vi "Arduino read multiple 10times resolution.vi"(6 "main loop iteration number":i32, 8 "arduino addresses in":T2, 10 "arduinos on?":bool) -> (1 "arduino addresses out":T2, 2 "unfiltered and mean of median filtered freq out":T1, 3 "arduinos on":bool)   [LabVIEW 2014]
uses:
  <vilib>/Analysis/baseanly.llb/Mean (DBL).vi
  <vilib>/Analysis/NI_AALBase.lvlib
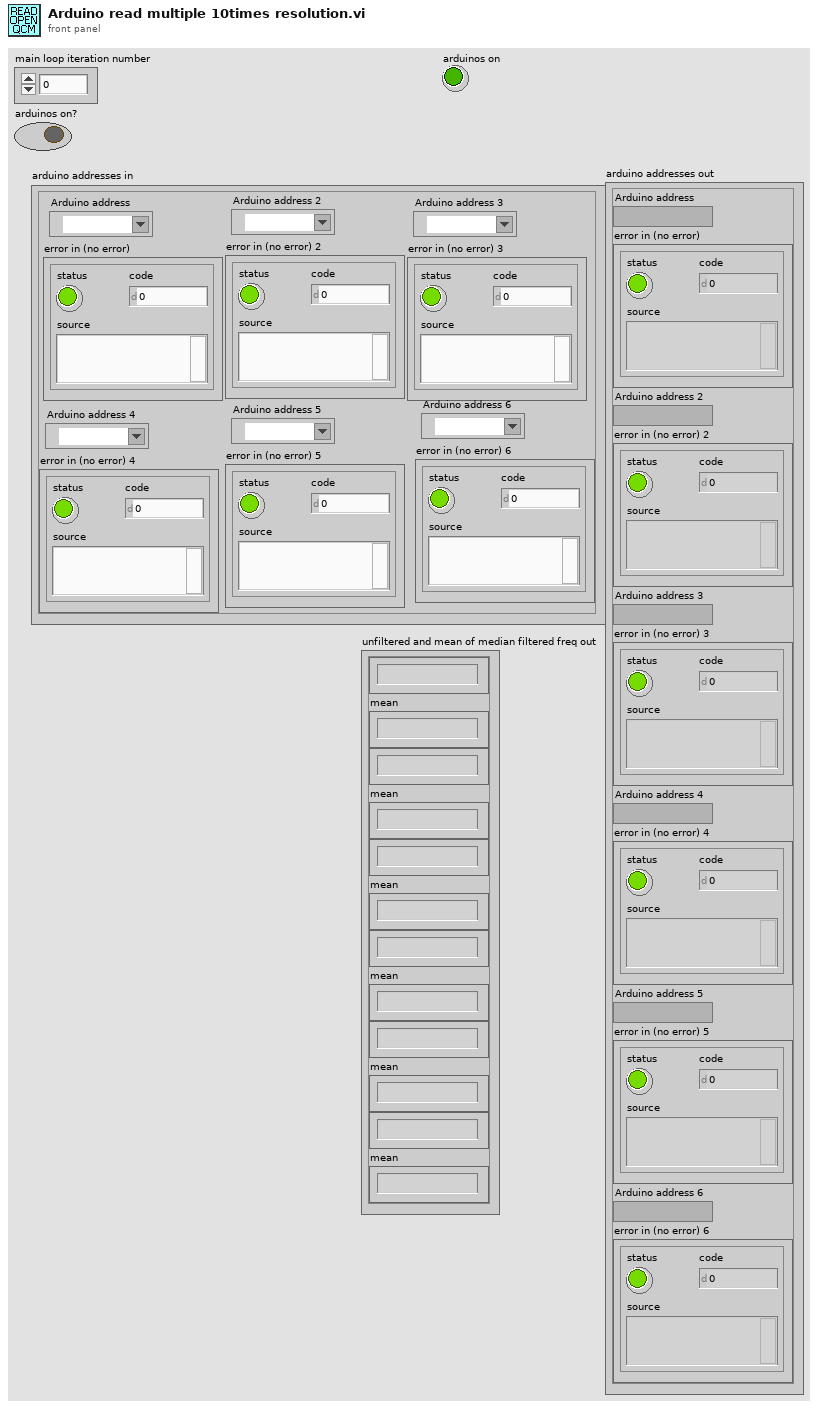
[diagram p1: front panel]
types:
  T1 = cluster{"String":string, "mean":string, "String":string, "mean":string, "String":string, "mean":string, "String":string, "mean":string, "String":string, "mean":string, "String":string, "mean":string}
  T2 = cluster{"Arduino address":refnum<visa-resource-name>, "error in (no error)":errorcluster, "Arduino address 2":refnum<visa-resource-name>, "error in (no error) 2":errorcluster, "Arduino address 3":refnum<visa-resource-name>, "error in (no error) 3":errorcluster, "Arduino address 4":refnum<visa-resource-name>, "error in (no error) 4":errorcluster, "Arduino address 5":refnum<visa-resource-name>, "error in (no error) 5":errorcluster, "Arduino address 6":refnum<visa-resource-name>, "error in (no error) 6":errorcluster}
  T3 = cluster{string, "mean":string, string, "mean":string, string, "mean":string, string, "mean":string, string, "mean":string, string, "mean":string}
  T4 = cluster{dbl, "mean":dbl, dbl, "mean":dbl, dbl, "mean":dbl, dbl, "mean":dbl, dbl, "mean":dbl, dbl, "mean":dbl}
  T5 = cluster{"Arduino address":refnum<visa-resource-name>, "error out":errorcluster, "Arduino address 2":refnum<visa-resource-name>, "error out":errorcluster, "Arduino address 3":refnum<visa-resource-name>, "error out":errorcluster, "Arduino address 4":refnum<visa-resource-name>, "error out":errorcluster, "Arduino address 5":refnum<visa-resource-name>, "error out":errorcluster, "Arduino address 6":refnum<visa-resource-name>, "error out":errorcluster}
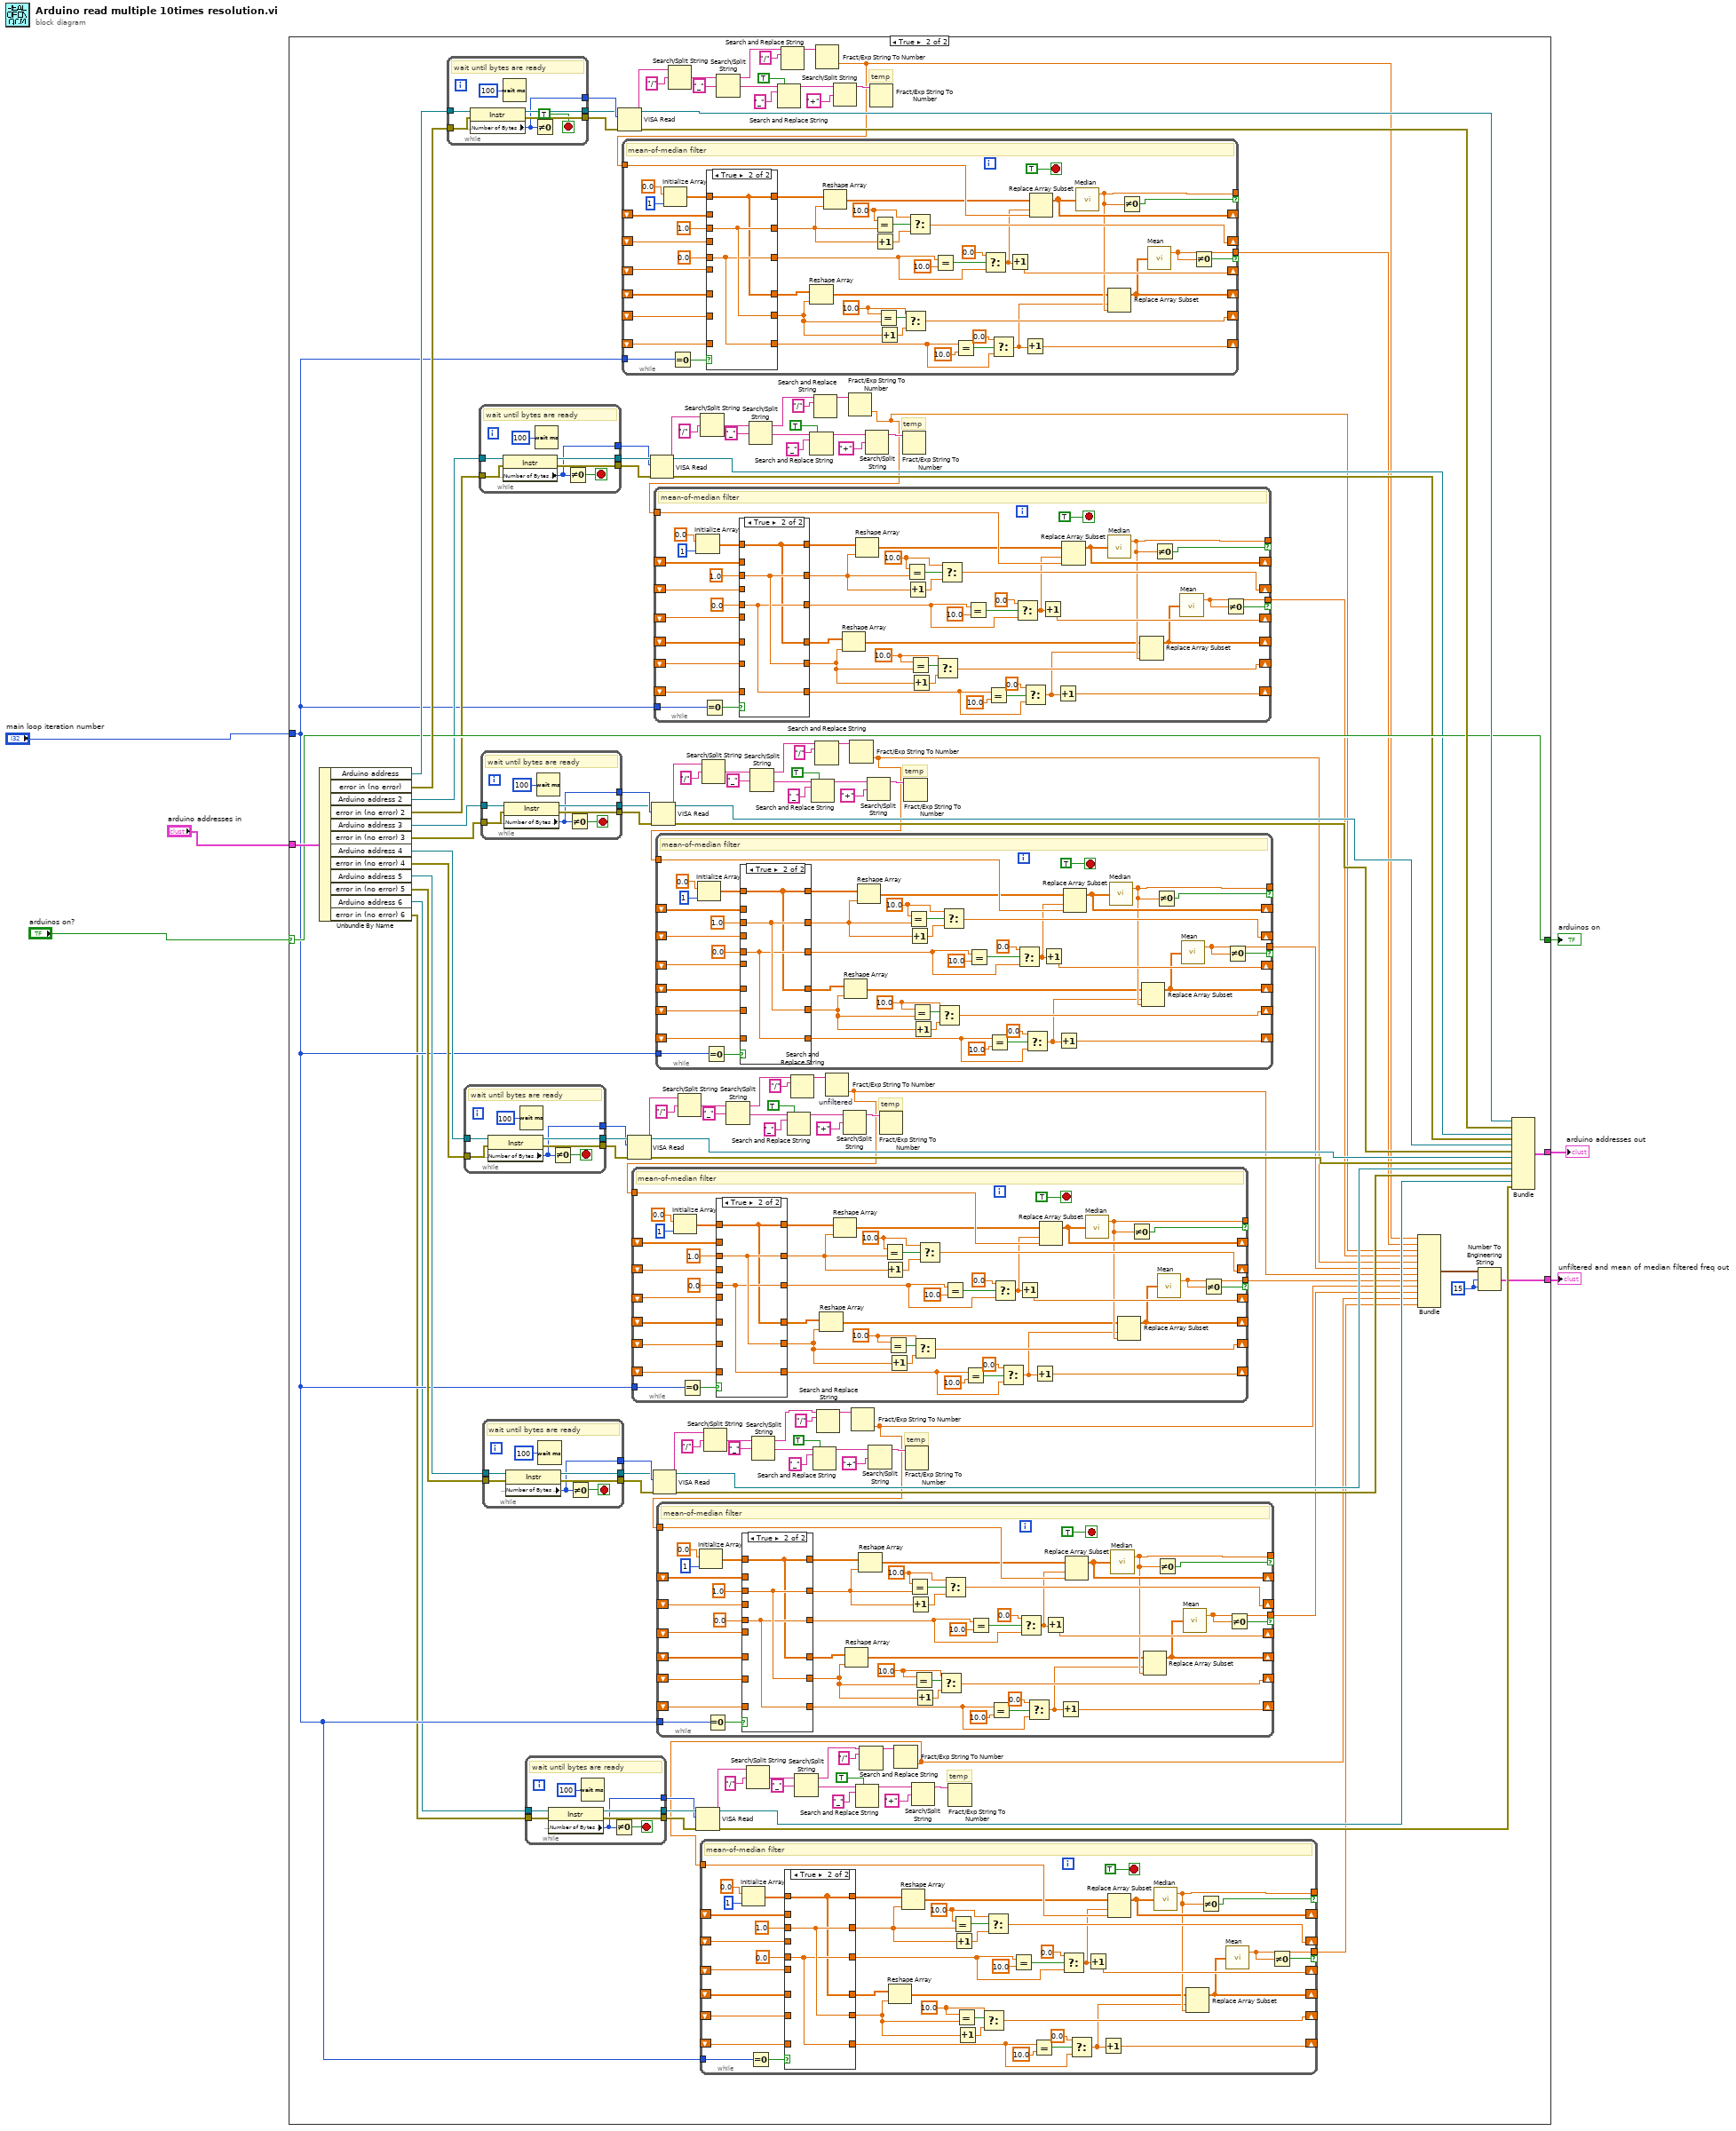
[diagram p0: block diagram]
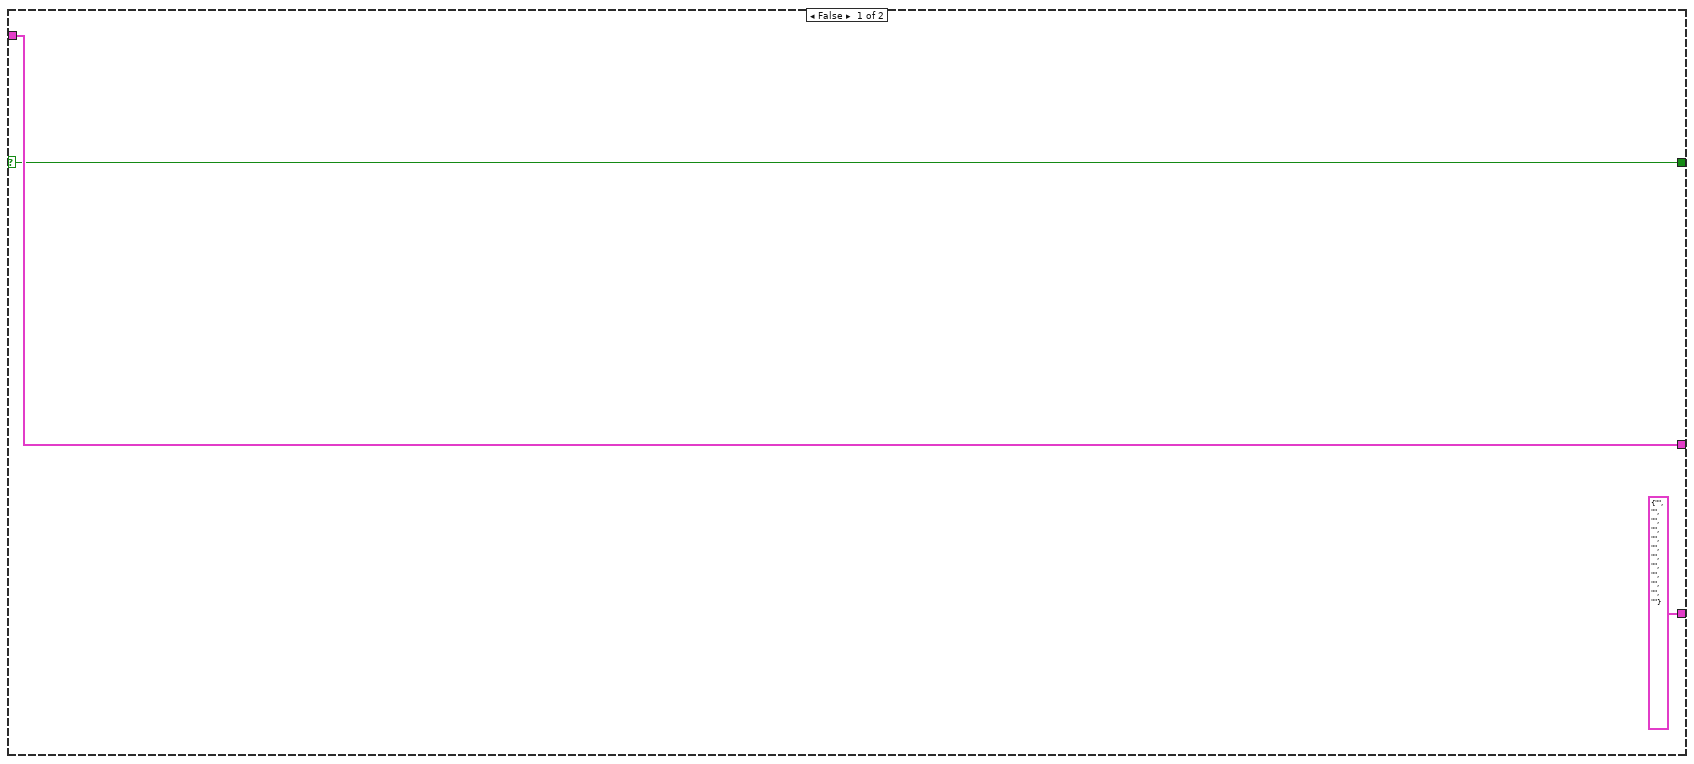
[diagram p2: hidden frame]
diagram:
  n1 = case shown="True" "arduinos on?" {
    selector: "arduinos on?" -> [w8 w126]
    tunnel: "main loop iteration number" -> [_ w31]
    tunnel: "arduino addresses in" -> [w9 w132]
    tunnel: [w9 w127] -> w2
    tunnel: [w8 w126] -> w3
    tunnel: [T3 {"", "mean"="", "", "mean"="", "", "mean"="", "", "mean"="", "", "mean"="", "", "mean"=""} w22] -> w1
    frame False {
    }
    frame True {
      w24 = i16 15 ("width (-)")
      # "temp"
      # "temp"
      # "temp"
      # "temp"
      # "temp"
      # "temp"
      n2 = Unbundle By Name(w132) -> ("Arduino address"=w131:refnum<visa-resource-name>, "error in (no error)"=w130:errorcluster, "Arduino address 2"=w109:refnum<visa-resource-name>, "error in (no error) 2"=w108:errorcluster, "Arduino address 3"=w89:refnum<visa-resource-name>, "error in (no error) 3"=w88:errorcluster, "Arduino address 4"=w69:refnum<visa-resource-name>, "error in (no error) 4"=w68:errorcluster, "Arduino address 5"=w51:refnum<visa-resource-name>, "error in (no error) 5"=w50:errorcluster, "Arduino address 6"=w30:refnum<visa-resource-name>, "error in (no error) 6"=w29:errorcluster)
      n3 = while {
        tunnel: w130 -> [w469]
        tunnel: w131 -> [w470]
        tunnel: [w468] -> w134
        tunnel: [w467] -> w133
        tunnel: [w466] -> w135
        stop <- TRUE stop-if-true
        # "wait until bytes are ready"
        n4 = property class="Instr"(reference=w470, error in=w469) -> (reference out=w467:refnum<visa-resource-name>, error out=w468:errorcluster, "Serial Settings:Number of Bytes at Serial Port"=w466:u32)
        n5 = Wait (ms)(milliseconds to wait=u32 100) -> ()  [unwired: 1 out]
        n6 = Not Equal To 0?(x=w466) -> ()  [unwired: 1 out]
      }
      n7 = while {
        tunnel: w68 -> [w280]
        tunnel: w69 -> [w281]
        tunnel: [w279] -> w84
        tunnel: [w278] -> w85
        tunnel: [w277] -> w83
        stop <- w275 stop-if-true
        # "wait until bytes are ready"
        n8 = property class="Instr"(reference=w281, error in=w280) -> (reference out=w278:refnum<visa-resource-name>, error out=w279:errorcluster, "Serial Settings:Number of Bytes at Serial Port"=w277:u32)
        n9 = Wait (ms)(milliseconds to wait=u32 100) -> ()  [unwired: 1 out]
        n10 = Not Equal To 0?(x=w277) -> (x != 0?=w275:bool)
      }
      n11 = while {
        tunnel: w108 -> [w406]
        tunnel: w109 -> [w407]
        tunnel: [w405] -> w124
        tunnel: [w404] -> w125
        tunnel: [w403] -> w123
        stop <- w401 stop-if-true
        # "wait until bytes are ready"
        n12 = property class="Instr"(reference=w407, error in=w406) -> (reference out=w404:refnum<visa-resource-name>, error out=w405:errorcluster, "Serial Settings:Number of Bytes at Serial Port"=w403:u32)
        n13 = Wait (ms)(milliseconds to wait=u32 100) -> ()  [unwired: 1 out]
        n14 = Not Equal To 0?(x=w403) -> (x != 0?=w401:bool)
      }
      n15 = while {
        tunnel: w88 -> [w343]
        tunnel: w89 -> [w344]
        tunnel: [w342] -> w91
        tunnel: [w341] -> w90
        tunnel: [w340] -> w92
        stop <- w338 stop-if-true
        # "wait until bytes are ready"
        n16 = property class="Instr"(reference=w344, error in=w343) -> (reference out=w341:refnum<visa-resource-name>, error out=w342:errorcluster, "Serial Settings:Number of Bytes at Serial Port"=w340:u32)
        n17 = Wait (ms)(milliseconds to wait=u32 100) -> ()  [unwired: 1 out]
        n18 = Not Equal To 0?(x=w340) -> (x != 0?=w338:bool)
      }
      n19 = while {
        tunnel: w51 -> [w218]
        tunnel: [w217] -> w53
        tunnel: [w216] -> w52
        tunnel: [w215] -> w54
        tunnel: w50 -> [w212]
        stop <- w213 stop-if-true
        # "wait until bytes are ready"
        n20 = property class="Instr"(reference=w218, error in=w212) -> (reference out=w216:refnum<visa-resource-name>, error out=w217:errorcluster, "Serial Settings:Number of Bytes at Serial Port"=w215:u32)
        n21 = Wait (ms)(milliseconds to wait=u32 100) -> ()  [unwired: 1 out]
        n22 = Not Equal To 0?(x=w215) -> (x != 0?=w213:bool)
      }
      n23 = while {
        tunnel: w30 -> [w155]
        tunnel: [w154] -> w46
        tunnel: [w153] -> w47
        tunnel: [w152] -> w45
        tunnel: w29 -> [w149]
        stop <- w150 stop-if-true
        # "wait until bytes are ready"
        n24 = property class="Instr"(reference=w155, error in=w149) -> (reference out=w153:refnum<visa-resource-name>, error out=w154:errorcluster, "Serial Settings:Number of Bytes at Serial Port"=w152:u32)
        n25 = Wait (ms)(milliseconds to wait=u32 100) -> ()  [unwired: 1 out]
        n26 = Not Equal To 0?(x=w152) -> (x != 0?=w150:bool)
      }
      n27 = VISA Read(VISA resource name=w133, byte count=w135, error in (no error)=w134) -> (VISA resource name out=w129:refnum<visa-resource-name>, read buffer=w148:string, error out=w128:errorcluster)  [unwired: 1 out]
      n28 = VISA Read(VISA resource name=w85, byte count=w83, error in (no error)=w84) -> (VISA resource name out=w67:refnum<visa-resource-name>, read buffer=w70:string, error out=w66:errorcluster)  [unwired: 1 out]
      n29 = VISA Read(VISA resource name=w125, byte count=w123, error in (no error)=w124) -> (VISA resource name out=w106:refnum<visa-resource-name>, read buffer=w110:string, error out=w107:errorcluster)  [unwired: 1 out]
      n30 = VISA Read(VISA resource name=w90, byte count=w92, error in (no error)=w91) -> (VISA resource name out=w87:refnum<visa-resource-name>, read buffer=w105:string, error out=w86:errorcluster)  [unwired: 1 out]
      n31 = VISA Read(VISA resource name=w52, byte count=w54, error in (no error)=w53) -> (VISA resource name out=w49:refnum<visa-resource-name>, read buffer=w65:string, error out=w48:errorcluster)  [unwired: 1 out]
      n32 = Search/Split String(string=w148, search string/char (-)="/") -> (match + rest of string=w141:string)  [unwired: 1 in, 2 out]
      n33 = Search/Split String(string=w70, search string/char (-)="/") -> (match + rest of string=w77:string)  [unwired: 1 in, 2 out]
      n34 = VISA Read(VISA resource name=w47, byte count=w45, error in (no error)=w46) -> (VISA resource name out=w26:refnum<visa-resource-name>, read buffer=w34:string, error out=w25:errorcluster)  [unwired: 1 out]
      n35 = Search/Split String(string=w110, search string/char (-)="/") -> (match + rest of string=w117:string)  [unwired: 1 in, 2 out]
      n36 = Search/Split String(string=w105, search string/char (-)="/") -> (match + rest of string=w98:string)  [unwired: 1 in, 2 out]
      n37 = Search/Split String(string=w65, search string/char (-)="/") -> (match + rest of string=w59:string)  [unwired: 1 in, 2 out]
      n38 = Search/Split String(string=w141, search string/char (-)="_") -> (substring before match=w147:string, match + rest of string=w142:string)  [unwired: 1 in, 1 out]
      n39 = Search/Split String(string=w77, search string/char (-)="_") -> (substring before match=w71:string, match + rest of string=w76:string)  [unwired: 1 in, 1 out]
      n40 = Search/Split String(string=w34, search string/char (-)="/") -> (match + rest of string=w40:string)  [unwired: 1 in, 2 out]
      n41 = Search/Split String(string=w117, search string/char (-)="_") -> (substring before match=w111:string, match + rest of string=w116:string)  [unwired: 1 in, 1 out]
      n42 = Search/Split String(string=w98, search string/char (-)="_") -> (substring before match=w104:string, match + rest of string=w99:string)  [unwired: 1 in, 1 out]
      n43 = Search/Split String(string=w59, search string/char (-)="_") -> (substring before match=w33:string, match + rest of string=w60:string)  [unwired: 1 in, 1 out]
      n44 = Search and Replace String(replace all?=TRUE ("replace all? (F)"), input string=w142, search string="_") -> (result string=w136:string)  [unwired: 5 in, 3 out]
      n45 = Search and Replace String(input string=w147, search string="/" ("replace string (\"\")")) -> (result string=w138:string)  [unwired: 6 in, 3 out]
      n46 = Search and Replace String(replace all?=TRUE ("replace all? (F)"), input string=w76, search string="_") -> (result string=w82:string)  [unwired: 5 in, 3 out]
      n47 = Search and Replace String(input string=w71, search string="/" ("replace string (\"\")")) -> (result string=w80:string)  [unwired: 6 in, 3 out]
      n48 = Search/Split String(string=w40, search string/char (-)="_") -> (substring before match=w28:string, match + rest of string=w39:string)  [unwired: 1 in, 1 out]
      n49 = Search and Replace String(replace all?=TRUE ("replace all? (F)"), input string=w116, search string="_") -> (result string=w122:string)  [unwired: 5 in, 3 out]
      n50 = Search and Replace String(replace all?=TRUE ("replace all? (F)"), input string=w99, search string="_") -> (result string=w93:string)  [unwired: 5 in, 3 out]
      n51 = Search and Replace String(replace all?=TRUE ("replace all? (F)"), input string=w60, search string="_") -> (result string=w55:string)  [unwired: 5 in, 3 out]
      n52 = Search and Replace String(input string=w111, search string="/" ("replace string (\"\")")) -> (result string=w120:string)  [unwired: 6 in, 3 out]
      n53 = Search and Replace String(input string=w104, search string="/" ("replace string (\"\")")) -> (result string=w95:string)  [unwired: 6 in, 3 out]
      n54 = Fract/Exp String To Number(string=w138) -> (number=w21:dbl)  [unwired: 3 in, 1 out]
      n55 = while {
        shift-right: [w509] -> _
        shift-left: _ -> [w487]
        shift-right: [w517] -> _
        shift-left: _ -> [w480]
        shift-right: [w506] -> _
        shift-left: _ -> [w477]
        shift-right: [w516] -> _
        shift-left: _ -> [w473]
        shift-right: [w515] -> _
        shift-left: _ -> [w484]
        tunnel: w21 -> [w512]
        tunnel: w31 -> [w489]
        tunnel: [w508] -> w15 if=w511
        tunnel: [w505] -> _ if=w504
        shift-right: [w507] -> _
        shift-left: _ -> [w475]
        stop <- TRUE stop-if-true
        w490 = 10.0 ("t")
        w482 = 10.0 ("y")
        # "mean-of-median filter"
        n56 = Initialize Array(0.0 ("element"), 1 ("dimension size")) -> (w478:dbl[])
        n57 = Equal To 0?(x=w489) -> (x = 0?=w488:bool)
        n58 = case shown="True" w488 {
          tunnel: w478 -> [_ w524]
          tunnel: w487 -> [w523 _]
          tunnel: [w523 w524] -> w486
          tunnel: 1.0 ("t") -> [_ w526]
          tunnel: w484 -> [w522 _]
          tunnel: [w522 w526] -> w483
          tunnel: 0.0 ("t") -> [_ w525]
          tunnel: [w521 w525] -> w479
          tunnel: w480 -> [w521 _]
          tunnel: [w520 w524] -> w476
          tunnel: w477 -> [w520 _]
          tunnel: [w519 w526] -> w474
          tunnel: w475 -> [w519 _]
          tunnel: w473 -> [w518 _]
          tunnel: [w518 w525] -> w472
          frame False {
          }
          frame True {
          }
        }
        n59 = Reshape Array(w476, w474) -> (w471:dbl[])
        n60 = Reshape Array(w486, w483) -> (w497:dbl[])
        n61 = Equal?(x=w482, y=w483) -> (x = y?=w496:bool)
        n62 = Increment(x=w483) -> (x+1=w495:dbl)
        n63 = Equal?(x=w490, y=w474) -> (x = y?=w493:bool)
        n64 = Increment(x=w474) -> (x+1=w492:dbl)
        n65 = Select(t=w490, s=w493, f=w492) -> (s? t:f=w507:dbl)
        n66 = Select(t=w482, s=w496, f=w495) -> (s? t:f=w515:dbl)
        n67 = Equal?(x=w479, y=10.0) -> (x = y?=w503:bool)
        n68 = Equal?(x=w472, y=10.0) -> (x = y?=w500:bool)
        n69 = Select(t=0.0, s=w503, f=w479) -> (s? t:f=w491:dbl)
        n70 = Select(t=0.0, s=w500, f=w472) -> (s? t:f=w499:dbl)
        n71 = Increment(x=w491) -> (x+1=w517:dbl)
        n72 = Increment(x=w499) -> (x+1=w516:dbl)
        n73 = Replace Array Subset(array=w497, new element=w512, index=w491) -> (w509:dbl[])
        n74 = call <vilib>:"Median.vi"("X"=w509) -> ("median"=w505:dbl)  [unwired: 1 out]
        n75 = Replace Array Subset(array=w471, new element=w505, index=w499) -> (w506:dbl[])
        n76 = Not Equal To 0?(x=w505) -> (x != 0?=w504:bool)
        n77 = call-poly <vilib>:"Mean.vi"("X"=w506) -> ("mean"=w508:dbl)  [unwired: 1 out]
        n78 = Not Equal To 0?(x=w508) -> (x != 0?=w511:bool)
      }
      n79 = Search and Replace String(input string=w33, search string="/" ("replace string (\"\")")) -> (result string=w32:string)  [unwired: 6 in, 3 out]
      n80 = Fract/Exp String To Number "unfiltered"(string=w80) -> (number=w18:dbl)  [unwired: 3 in, 1 out]
      n81 = while {
        shift-right: [w320] -> _
        shift-left: _ -> [w298]
        shift-right: [w328] -> _
        shift-left: _ -> [w291]
        shift-right: [w317] -> _
        shift-left: _ -> [w288]
        shift-right: [w327] -> _
        shift-left: _ -> [w284]
        shift-right: [w326] -> _
        shift-left: _ -> [w295]
        tunnel: w18 -> [w323]
        tunnel: w31 -> [w300]
        tunnel: [w319] -> w12 if=w322
        tunnel: [w316] -> _ if=w315
        shift-right: [w318] -> _
        shift-left: _ -> [w286]
        stop <- TRUE stop-if-true
        w301 = 10.0 ("t")
        w293 = 10.0 ("y")
        # "mean-of-median filter"
        n82 = Initialize Array(0.0 ("element"), 1 ("dimension size")) -> (w289:dbl[])
        n83 = Equal To 0?(x=w300) -> (x = 0?=w299:bool)
        n84 = case shown="True" w299 {
          tunnel: w289 -> [_ w335]
          tunnel: w298 -> [w334 _]
          tunnel: [w334 w335] -> w297
          tunnel: 1.0 ("t") -> [_ w337]
          tunnel: w295 -> [w333 _]
          tunnel: [w333 w337] -> w294
          tunnel: 0.0 ("t") -> [_ w336]
          tunnel: [w332 w336] -> w290
          tunnel: w291 -> [w332 _]
          tunnel: [w331 w335] -> w287
          tunnel: w288 -> [w331 _]
          tunnel: [w330 w337] -> w285
          tunnel: w286 -> [w330 _]
          tunnel: w284 -> [w329 _]
          tunnel: [w329 w336] -> w283
          frame False {
          }
          frame True {
          }
        }
        n85 = Reshape Array(w287, w285) -> (w282:dbl[])
        n86 = Reshape Array(w297, w294) -> (w308:dbl[])
        n87 = Equal?(x=w293, y=w294) -> (x = y?=w307:bool)
        n88 = Increment(x=w294) -> (x+1=w306:dbl)
        n89 = Equal?(x=w301, y=w285) -> (x = y?=w304:bool)
        n90 = Increment(x=w285) -> (x+1=w303:dbl)
        n91 = Select(t=w301, s=w304, f=w303) -> (s? t:f=w318:dbl)
        n92 = Select(t=w293, s=w307, f=w306) -> (s? t:f=w326:dbl)
        n93 = Equal?(x=w290, y=10.0) -> (x = y?=w314:bool)
        n94 = Equal?(x=w283, y=10.0) -> (x = y?=w311:bool)
        n95 = Select(t=0.0, s=w314, f=w290) -> (s? t:f=w302:dbl)
        n96 = Select(t=0.0, s=w311, f=w283) -> (s? t:f=w310:dbl)
        n97 = Increment(x=w302) -> (x+1=w328:dbl)
        n98 = Increment(x=w310) -> (x+1=w327:dbl)
        n99 = Replace Array Subset(array=w308, new element=w323, index=w302) -> (w320:dbl[])
        n100 = call <vilib>:"Median.vi"("X"=w320) -> ("median"=w316:dbl)  [unwired: 1 out]
        n101 = Replace Array Subset(array=w282, new element=w316, index=w310) -> (w317:dbl[])
        n102 = Not Equal To 0?(x=w316) -> (x != 0?=w315:bool)
        n103 = call-poly <vilib>:"Mean.vi"("X"=w317) -> ("mean"=w319:dbl)  [unwired: 1 out]
        n104 = Not Equal To 0?(x=w319) -> (x != 0?=w322:bool)
      }
      n105 = Search/Split String(string=w136, search string/char (-)="+") -> (substring before match=w145:string)  [unwired: 1 in, 2 out]
      n106 = Search/Split String(string=w82, search string/char (-)="+") -> (substring before match=w73:string)  [unwired: 1 in, 2 out]
      n107 = Fract/Exp String To Number(string=w120) -> (number=w20:dbl)  [unwired: 3 in, 1 out]
      n108 = while {
        shift-right: [w446] -> _
        shift-left: _ -> [w424]
        shift-right: [w454] -> _
        shift-left: _ -> [w417]
        shift-right: [w443] -> _
        shift-left: _ -> [w414]
        shift-right: [w453] -> _
        shift-left: _ -> [w410]
        shift-right: [w452] -> _
        shift-left: _ -> [w421]
        tunnel: w20 -> [w449]
        tunnel: w31 -> [w426]
        tunnel: [w445] -> w14 if=w448
        tunnel: [w442] -> _ if=w441
        shift-right: [w444] -> _
        shift-left: _ -> [w412]
        stop <- TRUE stop-if-true
        w427 = 10.0 ("t")
        w419 = 10.0 ("y")
        # "mean-of-median filter"
        n109 = Initialize Array(0.0 ("element"), 1 ("dimension size")) -> (w415:dbl[])
        n110 = Equal To 0?(x=w426) -> (x = 0?=w425:bool)
        n111 = case shown="True" w425 {
          tunnel: w415 -> [_ w461]
          tunnel: w424 -> [w460 _]
          tunnel: [w460 w461] -> w423
          tunnel: 1.0 ("t") -> [_ w463]
          tunnel: w421 -> [w459 _]
          tunnel: [w459 w463] -> w420
          tunnel: 0.0 ("t") -> [_ w462]
          tunnel: [w458 w462] -> w416
          tunnel: w417 -> [w458 _]
          tunnel: [w457 w461] -> w413
          tunnel: w414 -> [w457 _]
          tunnel: [w456 w463] -> w411
          tunnel: w412 -> [w456 _]
          tunnel: w410 -> [w455 _]
          tunnel: [w455 w462] -> w409
          frame False {
          }
          frame True {
          }
        }
        n112 = Reshape Array(w413, w411) -> (w408:dbl[])
        n113 = Reshape Array(w423, w420) -> (w434:dbl[])
        n114 = Equal?(x=w419, y=w420) -> (x = y?=w433:bool)
        n115 = Increment(x=w420) -> (x+1=w432:dbl)
        n116 = Equal?(x=w427, y=w411) -> (x = y?=w430:bool)
        n117 = Increment(x=w411) -> (x+1=w429:dbl)
        n118 = Select(t=w427, s=w430, f=w429) -> (s? t:f=w444:dbl)
        n119 = Select(t=w419, s=w433, f=w432) -> (s? t:f=w452:dbl)
        n120 = Equal?(x=w416, y=10.0) -> (x = y?=w440:bool)
        n121 = Equal?(x=w409, y=10.0) -> (x = y?=w437:bool)
        n122 = Select(t=0.0, s=w440, f=w416) -> (s? t:f=w428:dbl)
        n123 = Select(t=0.0, s=w437, f=w409) -> (s? t:f=w436:dbl)
        n124 = Increment(x=w428) -> (x+1=w454:dbl)
        n125 = Increment(x=w436) -> (x+1=w453:dbl)
        n126 = Replace Array Subset(array=w434, new element=w449, index=w428) -> (w446:dbl[])
        n127 = call <vilib>:"Median.vi"("X"=w446) -> ("median"=w442:dbl)  [unwired: 1 out]
        n128 = Replace Array Subset(array=w408, new element=w442, index=w436) -> (w443:dbl[])
        n129 = Not Equal To 0?(x=w442) -> (x != 0?=w441:bool)
        n130 = call-poly <vilib>:"Mean.vi"("X"=w443) -> ("mean"=w445:dbl)  [unwired: 1 out]
        n131 = Not Equal To 0?(x=w445) -> (x != 0?=w448:bool)
      }
      n132 = Fract/Exp String To Number(string=w95) -> (number=w19:dbl)  [unwired: 3 in, 1 out]
      n133 = while {
        shift-right: [w383] -> _
        shift-left: _ -> [w361]
        shift-right: [w391] -> _
        shift-left: _ -> [w354]
        shift-right: [w380] -> _
        shift-left: _ -> [w351]
        shift-right: [w390] -> _
        shift-left: _ -> [w347]
        shift-right: [w389] -> _
        shift-left: _ -> [w358]
        tunnel: w19 -> [w386]
        tunnel: w31 -> [w363]
        tunnel: [w382] -> w13 if=w385
        tunnel: [w379] -> _ if=w378
        shift-right: [w381] -> _
        shift-left: _ -> [w349]
        stop <- TRUE stop-if-true
        w364 = 10.0 ("t")
        w356 = 10.0 ("y")
        # "mean-of-median filter"
        n134 = Initialize Array(0.0 ("element"), 1 ("dimension size")) -> (w352:dbl[])
        n135 = Equal To 0?(x=w363) -> (x = 0?=w362:bool)
        n136 = case shown="True" w362 {
          tunnel: w352 -> [_ w398]
          tunnel: w361 -> [w397 _]
          tunnel: [w397 w398] -> w360
          tunnel: 1.0 ("t") -> [_ w400]
          tunnel: w358 -> [w396 _]
          tunnel: [w396 w400] -> w357
          tunnel: 0.0 ("t") -> [_ w399]
          tunnel: [w395 w399] -> w353
          tunnel: w354 -> [w395 _]
          tunnel: [w394 w398] -> w350
          tunnel: w351 -> [w394 _]
          tunnel: [w393 w400] -> w348
          tunnel: w349 -> [w393 _]
          tunnel: w347 -> [w392 _]
          tunnel: [w392 w399] -> w346
          frame False {
          }
          frame True {
          }
        }
        n137 = Reshape Array(w350, w348) -> (w345:dbl[])
        n138 = Reshape Array(w360, w357) -> (w371:dbl[])
        n139 = Equal?(x=w356, y=w357) -> (x = y?=w370:bool)
        n140 = Increment(x=w357) -> (x+1=w369:dbl)
        n141 = Equal?(x=w364, y=w348) -> (x = y?=w367:bool)
        n142 = Increment(x=w348) -> (x+1=w366:dbl)
        n143 = Select(t=w364, s=w367, f=w366) -> (s? t:f=w381:dbl)
        n144 = Select(t=w356, s=w370, f=w369) -> (s? t:f=w389:dbl)
        n145 = Equal?(x=w353, y=10.0) -> (x = y?=w377:bool)
        n146 = Equal?(x=w346, y=10.0) -> (x = y?=w374:bool)
        n147 = Select(t=0.0, s=w377, f=w353) -> (s? t:f=w365:dbl)
        n148 = Select(t=0.0, s=w374, f=w346) -> (s? t:f=w373:dbl)
        n149 = Increment(x=w365) -> (x+1=w391:dbl)
        n150 = Increment(x=w373) -> (x+1=w390:dbl)
        n151 = Replace Array Subset(array=w371, new element=w386, index=w365) -> (w383:dbl[])
        n152 = call <vilib>:"Median.vi"("X"=w383) -> ("median"=w379:dbl)  [unwired: 1 out]
        n153 = Replace Array Subset(array=w345, new element=w379, index=w373) -> (w380:dbl[])
        n154 = Not Equal To 0?(x=w379) -> (x != 0?=w378:bool)
        n155 = call-poly <vilib>:"Mean.vi"("X"=w380) -> ("mean"=w382:dbl)  [unwired: 1 out]
        n156 = Not Equal To 0?(x=w382) -> (x != 0?=w385:bool)
      }
      n157 = Fract/Exp String To Number(string=w32) -> (number=w17:dbl)  [unwired: 3 in, 1 out]
      n158 = while {
        shift-right: [w257] -> _
        shift-left: _ -> [w235]
        shift-right: [w265] -> _
        shift-left: _ -> [w228]
        shift-right: [w254] -> _
        shift-left: _ -> [w225]
        shift-right: [w264] -> _
        shift-left: _ -> [w221]
        shift-right: [w263] -> _
        shift-left: _ -> [w232]
        tunnel: w17 -> [w260]
        tunnel: w31 -> [w237]
        tunnel: [w256] -> w11 if=w259
        tunnel: [w253] -> _ if=w252
        shift-right: [w255] -> _
        shift-left: _ -> [w223]
        stop <- TRUE stop-if-true
        w238 = 10.0 ("t")
        w230 = 10.0 ("y")
        # "mean-of-median filter"
        n159 = Initialize Array(0.0 ("element"), 1 ("dimension size")) -> (w226:dbl[])
        n160 = Equal To 0?(x=w237) -> (x = 0?=w236:bool)
        n161 = case shown="True" w236 {
          tunnel: w226 -> [_ w272]
          tunnel: w235 -> [w271 _]
          tunnel: [w271 w272] -> w234
          tunnel: 1.0 ("t") -> [_ w274]
          tunnel: w232 -> [w270 _]
          tunnel: [w270 w274] -> w231
          tunnel: 0.0 ("t") -> [_ w273]
          tunnel: [w269 w273] -> w227
          tunnel: w228 -> [w269 _]
          tunnel: [w268 w272] -> w224
          tunnel: w225 -> [w268 _]
          tunnel: [w267 w274] -> w222
          tunnel: w223 -> [w267 _]
          tunnel: w221 -> [w266 _]
          tunnel: [w266 w273] -> w220
          frame False {
          }
          frame True {
          }
        }
        n162 = Reshape Array(w224, w222) -> (w219:dbl[])
        n163 = Reshape Array(w234, w231) -> (w245:dbl[])
        n164 = Equal?(x=w230, y=w231) -> (x = y?=w244:bool)
        n165 = Increment(x=w231) -> (x+1=w243:dbl)
        n166 = Equal?(x=w238, y=w222) -> (x = y?=w241:bool)
        n167 = Increment(x=w222) -> (x+1=w240:dbl)
        n168 = Select(t=w238, s=w241, f=w240) -> (s? t:f=w255:dbl)
        n169 = Select(t=w230, s=w244, f=w243) -> (s? t:f=w263:dbl)
        n170 = Equal?(x=w227, y=10.0) -> (x = y?=w251:bool)
        n171 = Equal?(x=w220, y=10.0) -> (x = y?=w248:bool)
        n172 = Select(t=0.0, s=w251, f=w227) -> (s? t:f=w239:dbl)
        n173 = Select(t=0.0, s=w248, f=w220) -> (s? t:f=w247:dbl)
        n174 = Increment(x=w239) -> (x+1=w265:dbl)
        n175 = Increment(x=w247) -> (x+1=w264:dbl)
        n176 = Replace Array Subset(array=w245, new element=w260, index=w239) -> (w257:dbl[])
        n177 = call <vilib>:"Median.vi"("X"=w257) -> ("median"=w253:dbl)  [unwired: 1 out]
        n178 = Replace Array Subset(array=w219, new element=w253, index=w247) -> (w254:dbl[])
        n179 = Not Equal To 0?(x=w253) -> (x != 0?=w252:bool)
        n180 = call-poly <vilib>:"Mean.vi"("X"=w254) -> ("mean"=w256:dbl)  [unwired: 1 out]
        n181 = Not Equal To 0?(x=w256) -> (x != 0?=w259:bool)
      }
      n182 = Search and Replace String(replace all?=TRUE ("replace all? (F)"), input string=w39, search string="_") -> (result string=w44:string)  [unwired: 5 in, 3 out]
      n183 = Search and Replace String(input string=w28, search string="/" ("replace string (\"\")")) -> (result string=w27:string)  [unwired: 6 in, 3 out]
      n184 = Search/Split String(string=w122, search string/char (-)="+") -> (substring before match=w113:string)  [unwired: 1 in, 2 out]
      n185 = Search/Split String(string=w93, search string/char (-)="+") -> (substring before match=w102:string)  [unwired: 1 in, 2 out]
      n186 = Search/Split String(string=w55, search string/char (-)="+") -> (substring before match=w63:string)  [unwired: 1 in, 2 out]
      n187 = Fract/Exp String To Number(string=w145) -> ()  [unwired: 3 in, 2 out]
      n188 = Fract/Exp String To Number(string=w73) -> ()  [unwired: 3 in, 2 out]
      n189 = Fract/Exp String To Number(string=w27) -> (number=w16:dbl)  [unwired: 3 in, 1 out]
      n190 = while {
        shift-right: [w194] -> _
        shift-left: _ -> [w172]
        shift-right: [w202] -> _
        shift-left: _ -> [w165]
        shift-right: [w191] -> _
        shift-left: _ -> [w162]
        shift-right: [w201] -> _
        shift-left: _ -> [w158]
        shift-right: [w200] -> _
        shift-left: _ -> [w169]
        tunnel: w16 -> [w197]
        tunnel: w31 -> [w174]
        tunnel: [w193] -> w10 if=w196
        tunnel: [w190] -> _ if=w189
        shift-right: [w192] -> _
        shift-left: _ -> [w160]
        stop <- TRUE stop-if-true
        w175 = 10.0 ("t")
        w167 = 10.0 ("y")
        # "mean-of-median filter"
        n191 = Initialize Array(0.0 ("element"), 1 ("dimension size")) -> (w163:dbl[])
        n192 = Equal To 0?(x=w174) -> (x = 0?=w173:bool)
        n193 = case shown="True" w173 {
          tunnel: w163 -> [_ w209]
          tunnel: w172 -> [w208 _]
          tunnel: [w208 w209] -> w171
          tunnel: 1.0 ("t") -> [_ w211]
          tunnel: w169 -> [w207 _]
          tunnel: [w207 w211] -> w168
          tunnel: 0.0 ("t") -> [_ w210]
          tunnel: [w206 w210] -> w164
          tunnel: w165 -> [w206 _]
          tunnel: [w205 w209] -> w161
          tunnel: w162 -> [w205 _]
          tunnel: [w204 w211] -> w159
          tunnel: w160 -> [w204 _]
          tunnel: w158 -> [w203 _]
          tunnel: [w203 w210] -> w157
          frame False {
          }
          frame True {
          }
        }
        n194 = Reshape Array(w161, w159) -> (w156:dbl[])
        n195 = Reshape Array(w171, w168) -> (w182:dbl[])
        n196 = Equal?(x=w167, y=w168) -> (x = y?=w181:bool)
        n197 = Increment(x=w168) -> (x+1=w180:dbl)
        n198 = Equal?(x=w175, y=w159) -> (x = y?=w178:bool)
        n199 = Increment(x=w159) -> (x+1=w177:dbl)
        n200 = Select(t=w175, s=w178, f=w177) -> (s? t:f=w192:dbl)
        n201 = Select(t=w167, s=w181, f=w180) -> (s? t:f=w200:dbl)
        n202 = Equal?(x=w164, y=10.0) -> (x = y?=w188:bool)
        n203 = Equal?(x=w157, y=10.0) -> (x = y?=w185:bool)
        n204 = Select(t=0.0, s=w188, f=w164) -> (s? t:f=w176:dbl)
        n205 = Select(t=0.0, s=w185, f=w157) -> (s? t:f=w184:dbl)
        n206 = Increment(x=w176) -> (x+1=w202:dbl)
        n207 = Increment(x=w184) -> (x+1=w201:dbl)
        n208 = Replace Array Subset(array=w182, new element=w197, index=w176) -> (w194:dbl[])
        n209 = call <vilib>:"Median.vi"("X"=w194) -> ("median"=w190:dbl)  [unwired: 1 out]
        n210 = Replace Array Subset(array=w156, new element=w190, index=w184) -> (w191:dbl[])
        n211 = Not Equal To 0?(x=w190) -> (x != 0?=w189:bool)
        n212 = call-poly <vilib>:"Mean.vi"("X"=w191) -> ("mean"=w193:dbl)  [unwired: 1 out]
        n213 = Not Equal To 0?(x=w193) -> (x != 0?=w196:bool)
      }
      n214 = Fract/Exp String To Number(string=w113) -> ()  [unwired: 3 in, 2 out]
      n215 = Fract/Exp String To Number(string=w102) -> ()  [unwired: 3 in, 2 out]
      n216 = Fract/Exp String To Number(string=w63) -> ()  [unwired: 3 in, 2 out]
      n217 = Search/Split String(string=w44, search string/char (-)="+") -> (substring before match=w36:string)  [unwired: 1 in, 2 out]
      n218 = Fract/Exp String To Number(string=w36) -> ()  [unwired: 3 in, 2 out]
      n219 = Bundle(w21, "mean"=w15, w20, "mean"=w14, w19, "mean"=w13, w18, "mean"=w12, w17, "mean"=w11, w16, "mean"=w10) -> (w23:T4)  [unwired: 1 in]
      n220 = Number To Engineering String(2:w24, 3:w24, 4:w23) -> (0:w22:T3)  [unwired: 1 in]
      n221 = Bundle("Arduino address"=w129, "error out"=w128, "Arduino address 2"=w106, "error out"=w107, "Arduino address 3"=w87, "error out"=w86, "Arduino address 4"=w67, "error out"=w66, "Arduino address 5"=w49, "error out"=w48, "Arduino address 6"=w26, "error out"=w25) -> (w127:T5)  [unwired: 1 in]
    }
  }
  "arduinos on" <- w3
  "arduino addresses out" <- w2
  "unfiltered and mean of median filtered freq out" <- w1
